vi "Add Header.vi"(8 "error in (no error)":errorcluster, 9 "value":string, 10 "header":string(combo)="User-Agent", 11 "HTTP Client Base in":refnum<class "HTTP Client Base.lvclass">) -> (0 "error out":errorcluster, 3 "HTTP Client Base out":refnum<class "HTTP Client Base.lvclass">)   [LabVIEW 2021, in "HTTP Client Base.lvclass"]
uses:
  HTTP Client Base.lvclass
  HTTP Client Base.lvclass/HTTP Client Base.ctl
  <vilib>/httpClient/LabVIEWHTTPClient.lvlib
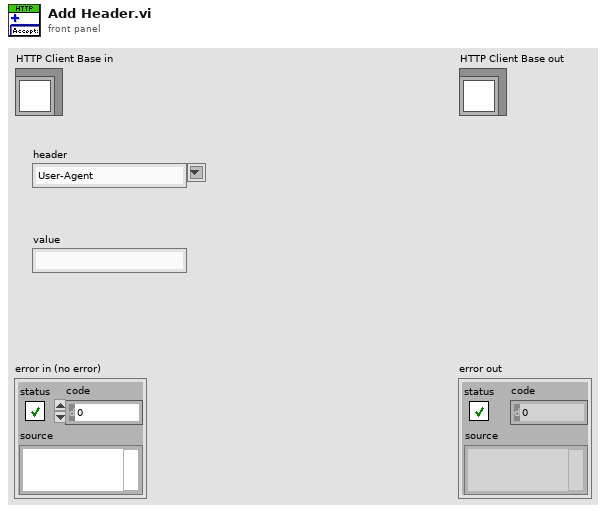
[diagram p1: front panel]
types:
  T1 = typedef "LabVIEWHTTPClient.lvlib/ClientHandle.ctl" = refnum<k1>
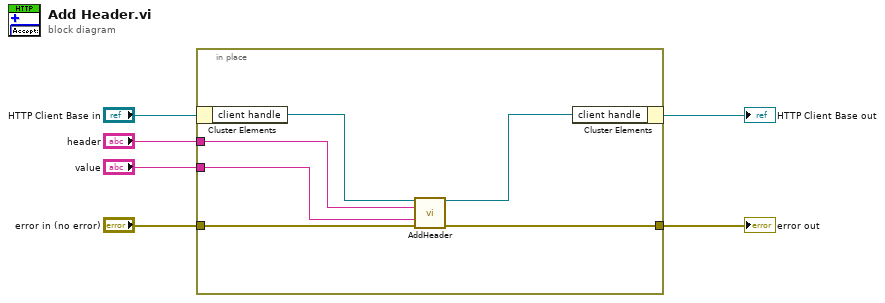
[diagram p0: block diagram]
diagram:
  n1 = in-place {
    in-place-border: "error in (no error)" -> [w11]
    in-place-border: [w10] -> w4
    in-place-border: "header" -> [w8]
    in-place-border: "value" -> [w7]
    n2 = in-place-cluster #1("HTTP Client Base in") -> ("client handle"=w12:T1)
    n3 = call <vilib>:"AddHeader.vi"("client handle"=w12, "header"=w8, "value"=w7, "error in (no error)"=w11) -> ("client handle out"=w9:T1, "error out"=w10:errorcluster)  [unwired: 10 in]
    n4 = in-place-cluster #1("client handle"=w9) -> (→"HTTP Client Base out":refnum<class "HTTP Client Base.lvclass">)
  }
  "error out" <- w4
